vi "TemperatureSweep.vi"(7 "Threshold":dbl(knob) scale=0.0..10.0, 8 "Stanford In":refnum<visa-resource-name>, 9 "Stanford Error":errorcluster, 10 "Keithley In":refnum<visa-resource-name>, 11 "Keithley Error":errorcluster) -> (0 "Stanford Out":refnum<visa-resource-name>, 1 "Stanford Err Out":errorcluster, 2 "Keithley Out":refnum<visa-resource-name>, 3 "Keithley Err Out":errorcluster)   [LabVIEW 2013]
uses:
  He3_Tlogger_Global 1.vi
  StopTempSweep.vi
  <vilib>/Utility/file.llb/Write To Spreadsheet File (DBL).vi
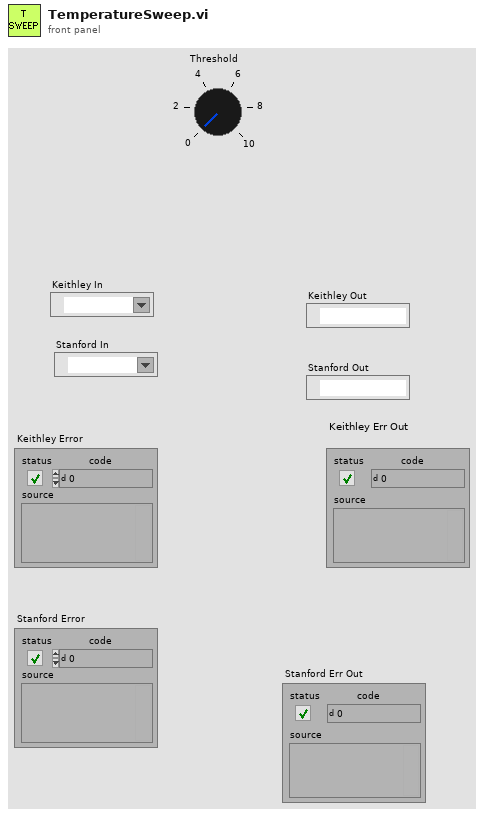
[diagram p1: front panel]
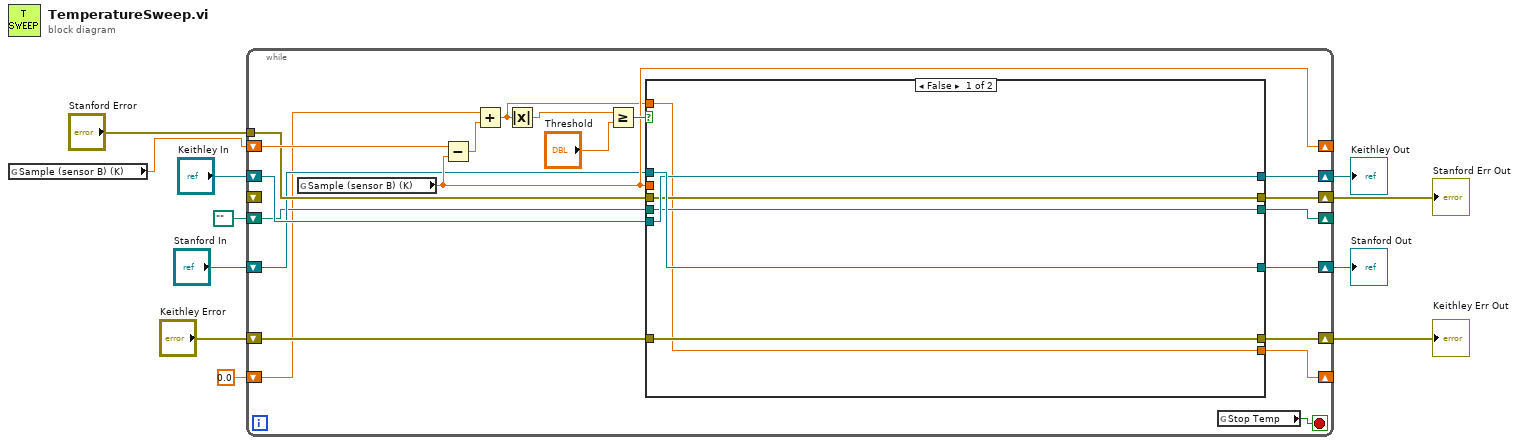
[diagram p0: block diagram]
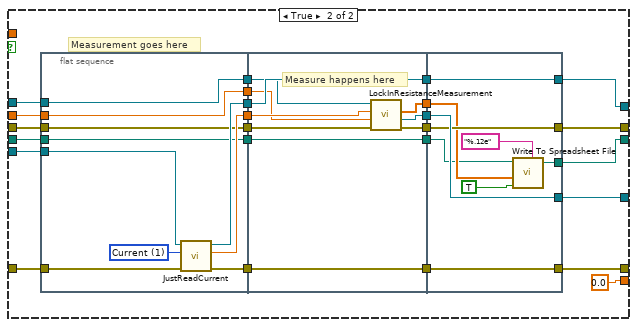
[diagram p2: hidden frame]
diagram:
  n1 = global read "He3_Tlogger_Global 1.vi" "Sample (sensor B) (K)"() -> (w11:dbl)
  n2 = while {
    shift-right: [w27] -> _
    shift-left: w11 -> [w31]
    tunnel: "Stanford Error" -> [w20]
    shift-right: [w26] -> w10
    shift-left: "Keithley In" -> [w24]
    shift-right: [w25] -> w9
    shift-left: "Stanford In" -> [w19]
    shift-right: [w23] -> w6
    shift-left: "Keithley Error" -> [w21]
    shift-right: [w22] -> w5
    shift-left: _ -> [_]
    shift-right: [w17] -> _
    shift-left: path "" ("new file path (Not A Path if cancelled)") -> [w16]
    shift-right: [w13] -> _
    shift-left: 0.0 -> [w15]
    stop <- w18 stop-if-true
    n3 = global read "He3_Tlogger_Global 1.vi" "Sample (sensor B) (K)"() -> (w27:dbl)
    n4 = Subtract(x=w31, y=w27) -> (x-y=w14:dbl)
    n5 = Add(x=w15, y=w14) -> (x+y=w12:dbl)
    n6 = Absolute Value(x=w12) -> (abs(x)=w30:dbl)
    n7 = Greater Or Equal?(x=w30, y="Threshold") -> (x >= y?=w28:bool)
    n8 = case shown="False" w28 {
      tunnel: w27 -> [_ w50]
      tunnel: [w36 w55] -> w26
      tunnel: [w37 w54] -> w25
      tunnel: w24 -> [w36 w53]
      tunnel: [w35 w52] -> w23
      tunnel: [w34 w51] -> w22
      tunnel: w21 -> [w35 w48]
      tunnel: w20 -> [w34 w47]
      tunnel: w19 -> [w37 w45]
      tunnel: [w33 w42] -> w17
      tunnel: w16 -> [w33 w39]
      tunnel: [w32 0.0] -> w13
      tunnel: w12 -> [w32 _]
      frame False {
      }
      frame True {
        # "Measurement goes here"
        n9 = flat-sequence {
          tunnel: [w72] -> w58
          tunnel: [w70] -> w57
          tunnel: [w71] -> w56
          tunnel: w53 -> [w69]
          tunnel: w50 -> [w68]
          tunnel: [w68] -> w49
          tunnel: w48 -> [w67]
          tunnel: w47 -> [w66]
          tunnel: [w66] -> w46
          tunnel: w45 -> [w65]
          tunnel: [w65] -> w44
          tunnel: w39 -> [w63]
          tunnel: [w63] -> w41
          tunnel: w58 -> [w82]
          tunnel: w57 -> [w80]
          tunnel: w56 -> [w81]
          tunnel: [w82] -> w62
          tunnel: [w81] -> w61
          tunnel: [w79] -> w60
          tunnel: [w78] -> w59
          tunnel: w49 -> [w77]
          tunnel: w46 -> [w76]
          tunnel: w44 -> [w75]
          tunnel: [w74] -> w43
          tunnel: w41 -> [w73]
          tunnel: [w73] -> w40
          tunnel: [w90] -> w52
          tunnel: [w91] -> w55
          tunnel: w62 -> [w91]
          tunnel: w61 -> [w90]
          tunnel: w60 -> [w89]
          tunnel: [w89] -> w54
          tunnel: [w88] -> w51
          tunnel: w59 -> [w88]
          tunnel: w43 -> [w86]
          tunnel: [w84] -> w42
          tunnel: w40 -> [w83]
          frame #0 {
            w64 = u16 1 items=["Volts", "Current", "Resistance"] ("Function (0: Volts)")
            n10 = call "JustReadCurrent.vi"("error in (no error)"=w67, "Function (0: Volts)"=w64, "Keithley In"=w69) -> ("error out"=w71:errorcluster, "Measured Current"=w70:dbl, "Keithley Out"=w72:refnum<visa-resource-name>)  [unwired: 6 in]
          }
          frame #1 {
            # "Measure happens here"
            n11 = call "LockInResistanceMeasurement.vi"("Stanford Error In"=w76, "Temperature"=w77, "Keithley Current"=w80, "Stanford ID"=w75) -> ("error out"=w78:errorcluster, "Stanford ID"=w79:refnum<visa-resource-name>, "Data Array"=w74:dbl[])  [unwired: 3 in, 1 out]
          }
          frame #2 {
            n12 = call-poly <vilib>:"Write To Spreadsheet File.vi"("format (%.3f)"="%.12e", "append to file? (new file:F)"=TRUE, "1D data"=w86, "file path (dialog if empty)"=w83) -> ("new file path (Not A Path if cancelled)"=w84:path)  [unwired: 4 in]
          }
        }
      }
    }
    n13 = global read "StopTempSweep.vi" "Stop Temp"() -> (w18:bool)
  }
  "Stanford Out" <- w9
  "Keithley Out" <- w10
  "Stanford Err Out" <- w5
  "Keithley Err Out" <- w6
